vi "Connector Pane Initialization.vi"(8 "error in (no error)":errorcluster, 11 "Data in":T1={"Class"={"Ants"=refnum, "Layer"=refnum, "Templates"=refnum, "Icon"=refnum, "Glyph"=refnum, "Settings"=refnum, "Tools"=refnum, "History"=refnum}, "Ref"={"Add Layer"=refnum, "Remove Layer"=refnum, "Line Text"=[], "Body Text Spec"=refnum, "DNL_Font"=refnum, "glyph path str"=refnum, "templates path str"=refnum, "Arrow Up"=refnum, "Arrow Down"=refnum, "IE VI Ref"=refnum, "Glyphs tree"=refnum, "Templates tree"=refnum, "Layer Icon Text"=refnum, "Layer Template"=refnum, "Body Text"=refnum, "Search Templates"=refnum, "TextMarker"=refnum, "Tab Control"=refnum, "Search Glyphs"=refnum, "Line Color"=refnum, "DNL_Glyphs []"=refnum, "Fill Color"=refnum, "Tools"=refnum, "Icon"=refnum, "Preview"=refnum, "Ants"=refnum, "Terminals"=refnum, "menu reference"=refnum, "LayerNames"=[], "GlyphLoadAnimation"=refnum, "TemplateLoadAnimation"=refnum, "refreshGlyphs"=refnum, "refreshTemplates"=refnum}, "Support"={"AntsRect"={"left"=0, "top"=0, "right"=0, "bottom"=0}, "Mouse Move Coords"={"Horizontal"=0, "Vertical"=0}, "Mouse Down Coords"={"Horizontal"=0, "Vertical"=0}, "Temp Coord"={"Horizontal"=0, "Vertical"=0}, "Action"=enum."Default", "Edge Color"=4914962, "Fill Color"=16860, "Mouse Down?"=FALSE, "Draft Mode?"=FALSE, "Temp Icon"=bytes[3102], "CTRL Pressed"=FALSE, "Move Selection?"=FALSE, "AntsRect Orig"={"left"=0, "top"=0, "right"=0, "bottom"=0}, "Text"="", "TM Set?"=FALSE, "Mouse inside icon?"=FALSE, "Tool (old value)"=0, "Pencil Move Color"=0, "Swap Colors?"=FALSE, "Shift pressed?"=FALSE}}) -> (0 "error out":errorcluster, 3 "Data out":T1={"Class"={"Ants"=refnum, "Layer"=refnum, "Templates"=refnum, "Icon"=refnum, "Glyph"=refnum, "Settings"=refnum, "Tools"=refnum, "History"=refnum}, "Ref"={"Add Layer"=refnum, "Remove Layer"=refnum, "Line Text"=[], "Body Text Spec"=refnum, "DNL_Font"=refnum, "glyph path str"=refnum, "templates path str"=refnum, "Arrow Up"=refnum, "Arrow Down"=refnum, "IE VI Ref"=refnum, "Glyphs tree"=refnum, "Templates tree"=refnum, "Layer Icon Text"=refnum, "Layer Template"=refnum, "Body Text"=refnum, "Search Templates"=refnum, "TextMarker"=refnum, "Tab Control"=refnum, "Search Glyphs"=refnum, "Line Color"=refnum, "DNL_Glyphs []"=refnum, "Fill Color"=refnum, "Tools"=refnum, "Icon"=refnum, "Preview"=refnum, "Ants"=refnum, "Terminals"=refnum, "menu reference"=refnum, "LayerNames"=[], "GlyphLoadAnimation"=refnum, "TemplateLoadAnimation"=refnum, "refreshGlyphs"=refnum, "refreshTemplates"=refnum}, "Support"={"AntsRect"={"left"=0, "top"=0, "right"=0, "bottom"=0}, "Mouse Move Coords"={"Horizontal"=0, "Vertical"=0}, "Mouse Down Coords"={"Horizontal"=0, "Vertical"=0}, "Temp Coord"={"Horizontal"=0, "Vertical"=0}, "Action"=enum."Default", "Edge Color"=4914962, "Fill Color"=16860, "Mouse Down?"=FALSE, "Draft Mode?"=FALSE, "Temp Icon"=bytes[3102], "CTRL Pressed"=FALSE, "Move Selection?"=FALSE, "AntsRect Orig"={"left"=0, "top"=0, "right"=0, "bottom"=0}, "Text"="", "TM Set?"=FALSE, "Mouse inside icon?"=FALSE, "Tool (old value)"=0, "Pencil Move Color"=0, "Swap Colors?"=FALSE, "Shift pressed?"=FALSE}})   [LabVIEW 2020]
uses:
  Class/Ants/Ants.lvclass
  Class/FakedArray/FakedArray.lvclass
  vi.lib/LabVIEW Icon API/lv_icon/Classes/Icon/Icon.lvclass
  Class/Icon Library/Glyph.lvclass
  Class/Settings/Settings.lvclass
  Class/Tools/Tools Paint.lvclass
  <vilib>/Utility/miscctls.llb/LVRectTypeDef.ctl
  <vilib>/Utility/miscctls.llb/LVPoint32TypeDef.ctl
  Controls/SupportClass_Action.ctl
  vi.lib/LabVIEW Icon API/lv_icon/Controls/IEColor.ctl
  Controls/Support Cluster.ctl
  lv_icon.lvlib
  Controls/References Cluster.ctl
  Controls/IE Classes.ctl
  Controls/Global Data.ctl
  History/History/History.lvclass
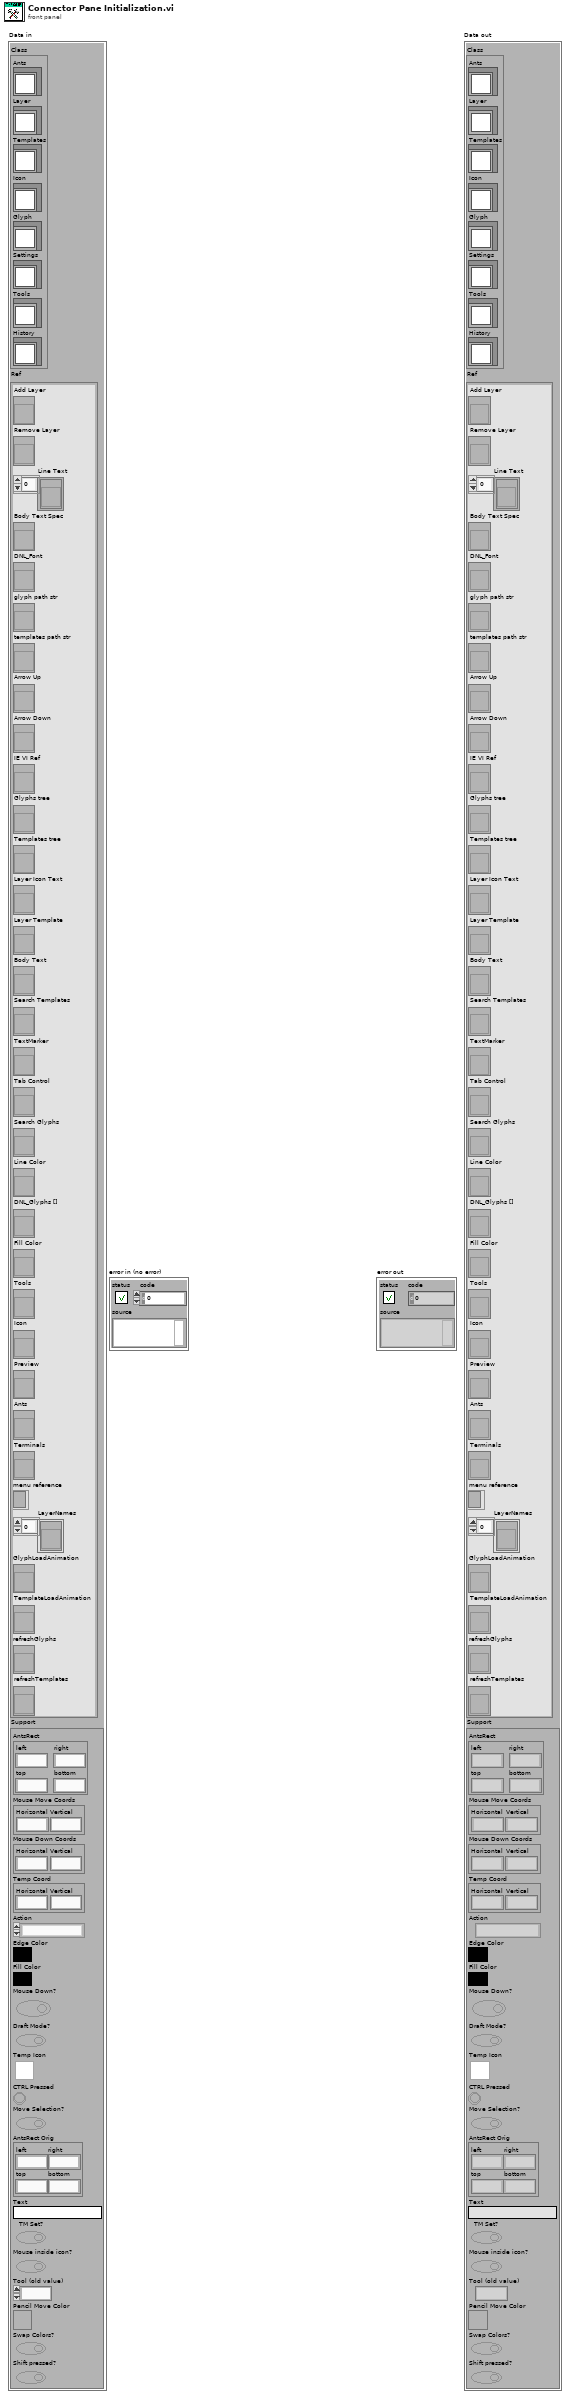
[diagram p1: front panel]
types:
  T1 = typedef "lv_icon.lvlib/Global Data.ctl" = cluster{"Class":T2, "Ref":T3, "Support":T4}
  T2 = typedef "lv_icon.lvlib/IE Classes.ctl" = cluster{"Ants":refnum<class "Ants.lvclass">, "Layer":refnum<class "FakedArray.lvclass">, "Templates":refnum<class "FakedArray.lvclass">, "Icon":refnum<class "Icon.lvclass">, "Glyph":refnum<class "Glyph.lvclass">, "Settings":refnum<class "Settings.lvclass">, "Tools":refnum<class "Tools Paint.lvclass">, "History":refnum<class "History.lvclass">}
  T3 = typedef "lv_icon.lvlib/References Cluster.ctl" = cluster{"Add Layer":refnum<vi>, "Remove Layer":refnum<vi>, "Line Text":refnum<vi>[], "Body Text Spec":refnum<vi>, "DNL_Font":refnum<vi>, "glyph path str":refnum<vi>, "templates path str":refnum<vi>, "Arrow Up":refnum<vi>, "Arrow Down":refnum<vi>, "IE VI Ref":refnum<vi>, "Glyphs tree":refnum<vi>, "Templates tree":refnum<vi>, "Layer Icon Text":refnum<vi>, "Layer Template":refnum<vi>, "Body Text":refnum<vi>, "Search Templates":refnum<vi>, "TextMarker":refnum<vi>, "Tab Control":refnum<vi>, "Search Glyphs":refnum<vi>, "Line Color":refnum<vi>, "DNL_Glyphs []":refnum<vi>, "Fill Color":refnum<vi>, "Tools":refnum<vi>, "Icon":refnum<vi>, "Preview":refnum<vi>, "Ants":refnum<vi>, "Terminals":refnum<vi>, "menu reference":refnum<k9>, "LayerNames":refnum<vi>[], "GlyphLoadAnimation":refnum<vi>, "TemplateLoadAnimation":refnum<vi>, "refreshGlyphs":refnum<vi>, "refreshTemplates":refnum<vi>}
  T4 = typedef "lv_icon.lvlib/Support Cluster.ctl" = cluster{"AntsRect":cluster{"left":i16, "top":i16, "right":i16, "bottom":i16}, "Mouse Move Coords":T5, "Mouse Down Coords":T5, "Temp Coord":T5, "Action":T6, "Edge Color":T7, "Fill Color":T7, "Mouse Down?":bool, "Draft Mode?":bool, "Temp Icon":picture, "CTRL Pressed":bool, "Move Selection?":bool, "AntsRect Orig":cluster{"left":i16, "top":i16, "right":i16, "bottom":i16}, "Text":string, "TM Set?":bool, "Mouse inside icon?":bool, "Tool (old value)":u32, "Pencil Move Color":u32, "Swap Colors?":bool, "Shift pressed?":bool}
  T5 = typedef "LVPoint32TypeDef.ctl" = cluster{"Horizontal":i32, "Vertical":i32}
  T6 = typedef "SupportClass_Action.ctl" = enum16{"Default", "Move Selection", "Glyph Library", "Tool"}
  T7 = typedef "IEColor.ctl" = u32
  T8 = typedef "LVRectTypeDef.ctl" = cluster{"Left":i16, "Top":i16, "Right":i16, "Bottom":i16}
  T9 = typedef "Who Invoked Icon Editor.ctl" = cluster{"Icon Editor Invoker Type":T10, "App Refnum of Invoker":refnum<vi>, "Qualified Name of Invoker":string, "Path to Invoker":path}
  T10 = typedef "Icon Editor Invoker Type.ctl" = enum32{"Unknown Icon Source", "VI Icon", "Library Icon (any library type)", "Palette icon", "Icon from App Method"}
  T11 = enum32{"invalid VI type", "Standard VI", "Control VI", "Global VI", "Polymorphic VI", "Configuration VI", "SubSystem", "Facade VI", "Method VI", "Statechart Diagram VI"}
  T12 = typedef "imagedata.ctl" = cluster{"image type":i32, "image depth":i32, "image":u8[], "mask":u8[], "colors":u32[], "Rectangle":cluster{"left":i16, "top":i16, "right":i16, "bottom":i16}}
  T13 = typedef "lv_icon.lvlib/INI Data.ctl" = cluster{"Show Terminals?":bool, "Text":cluster{"Font":T14, "Alignment":T15, "Size":T16}, "3rd party Templates":cluster{"Store 3rd party Templates?":bool, "Folder Name":string}, "Merge user layers on commit":bool, "Body Text":T17, "Fill Color":T7, "Edge Color":T7, "Tab":u16, "Tool":T18, "Disable Layers?":bool}
  T14 = typedef "Font.ctl" = string
  T15 = typedef "Alignment.ctl" = u16
  T16 = typedef "Font Size.ctl" = u8
  T17 = typedef "BodyText.ctl" = cluster{"Line 1 text":string, "Line 2 text":string, "Line 3 text":string, "Line 4 text":string, "Line 1 color":u32, "Line 2 color":u32, "Line 3 color":u32, "Line 4 color":u32, "Body Text Spec":cluster{"Font":T14, "Alignment":T15, "Size":u8}, "Center text vertically":bool, "Capitalize Text":bool}
  T18 = typedef "Tools.ctl" = enum32{"Pencil", "Line", "Dropper", "Fill", "Rectangle", "Filled Rectangle", "Ellipse", "Filled Ellipse", "Eraser", "Text", "Select", "Move"}
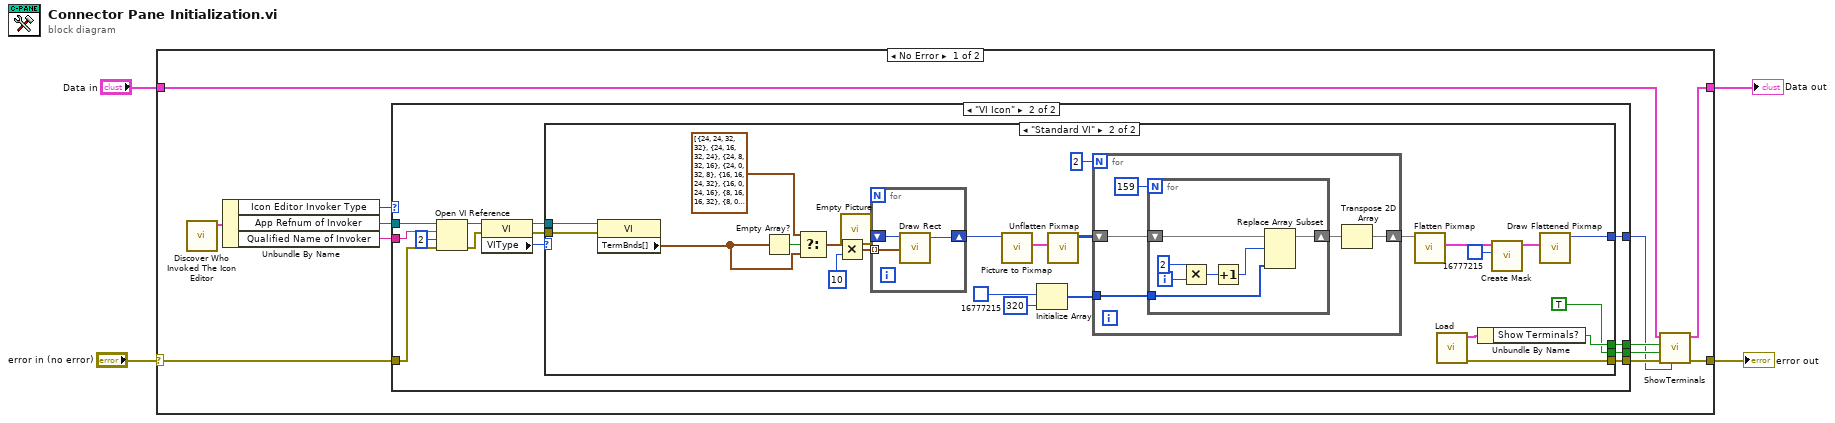
[diagram p0: block diagram]
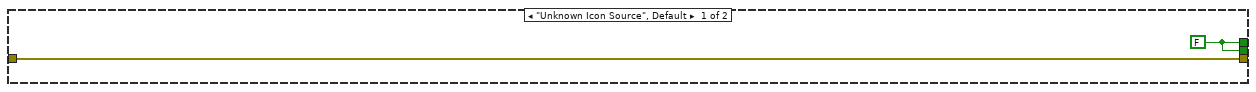
[diagram p2: hidden frame]
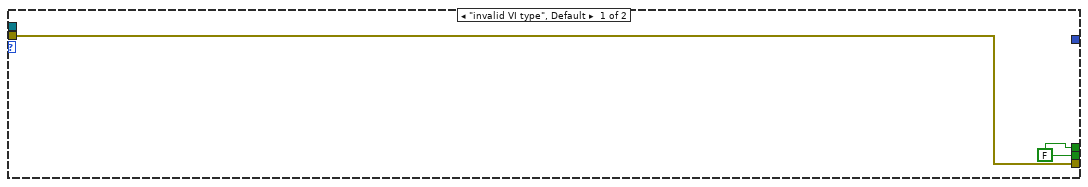
[diagram p3: hidden frame]
diagram:
  n1 = case shown="No Error" "error in (no error)" {
    selector: "error in (no error)" -> [w11 w75]
    tunnel: [w16 w75] -> w3
    tunnel: "Data in" -> [w7 w74]
    tunnel: [w6 w74] -> w1
    frame No Error {
      n2 = call <resource>:"Discover Who Invoked The Icon Editor.vi"() -> ("Who Invoked The Icon Editor?"=w14:T9)  [unwired: 11 out]
      n3 = Unbundle By Name(w14) -> ("Icon Editor Invoker Type"=w9:T10, "App Refnum of Invoker"=w13:refnum<vi>, "Qualified Name of Invoker"=w12:string)
      n4 = case shown="\"VI Icon\"" w9 {
        tunnel: [w18 w31] -> w15
        tunnel: w13 -> [_ w30]
        tunnel: w12 -> [_ w29]
        tunnel: w11 -> [w17 w28]
        tunnel: [w17 w27] -> w10
        tunnel: [w18 w26] -> w8
        tunnel: [_ w20] -> w5
        frame "Unknown Icon Source", Default {
          w18 = FALSE
        }
        frame "VI Icon" {
          n5 = Open VI Reference(application reference (local)=w30, vi path=w29, options=2, error in (no error)=w28) -> (vi reference=w22:refnum<vi>, error out=w23:errorcluster)  [unwired: 2 out]
          n6 = property class="VI"(reference=w22, error in=w23) -> (reference out=w25:refnum<vi>, error out=w24:errorcluster, "VIType"=w21:T11)
          n7 = case shown="\"Standard VI\"" w21 {
            tunnel: [w32 w57] -> w31
            tunnel: [w33 w56] -> w27
            tunnel: [w32 TRUE] -> w26
            tunnel: w25 -> [_ w36]
            tunnel: w24 -> [w33 w35]
            tunnel: [_ w43] -> w20
            frame "invalid VI type", Default {
              w32 = FALSE
            }
            frame "Standard VI" {
              n8 = property class="VI"(reference=w36, error in=w35) -> ("TermBnds[]"=w34:T8[])  [unwired: 2 out]
              n9 = Empty Array?(array=w34) -> (empty?=w42:bool)
              n10 = Select(t=T8[] [{"Left"=24, "Top"=24, "Right"=32, "Bottom"=32}, {"Left"=24, "Top"=16, "Right"=32, "Bottom"=24}, {"Left"=24, "Top"=8, "Right"=32, "Bottom"=16}, {"Left"=24, "Top"=0, "Right"=32, "Bottom"=8}, {"Left"=16, "Top"=16, "Right"=24, "Bottom"=32}, {"Left"=16, "Top"=0, "Right"=24, "Bottom"=16}, {"Left"=8, "Top"=16, "Right"=16, "Bottom"=32}, {"Left"=8, "Top"=0, "Right"=16, "Bottom"=16}, {"Left"=0, "Top"=24, "Right"=8, "Bottom"=32}, {"Left"=0, "Top"=16, "Right"=8, "Bottom"=24}, {"Left"=0, "Top"=8, "Right"=8, "Bottom"=16}, {"Left"=0, "Top"=0, "Right"=8, "Bottom"=8}] ("Terminal Bounds[]"), s=w42, f=w34) -> (s? t:f=w41:T8[])
              n11 = Multiply(x=w41, y=i16 10) -> (x*y=w45:T8[])
              n12 = call "Empty Picture"() -> ("empty picture"=w46:picture)
              n13 = for {
                tunnel: w45 -> [w73] mode=indexing
                shift-right: [w72] -> w47
                shift-left: w46 -> [w71]
                n14 = call <vilib>:"Draw Rect.vi"("picture"=w71, "rect"=w73) -> ("new picture"=w72:picture)  [unwired: 7 in]
              }
              n15 = call <vilib>:"Picture to Pixmap.vi"("picture"=w47) -> ("image data"=w48:T12)  [unwired: 9 in, 1 out]
              n16 = Initialize Array(u32 16777215, 320 ("dimension size")) -> (w53:u32[])
              n17 = call <vilib>:"Unflatten Pixmap.vi"("image data"=w48) -> ("24-bit pixmap"=w49:u32[][])  [unwired: 4 in, 6 out]
              n18 = for {
                N: 2 -> [_]
                shift-right: [w61] -> w54
                shift-left: w49 -> [w63]
                tunnel: w53 -> [w59]
                n19 = for {
                  N: 159 -> [_]
                  shift-right: [w65] -> w62
                  shift-left: w63 -> [w70]
                  tunnel: w59 -> [w64]
                  i -> [w69]
                  n20 = Multiply(x=2, y=w69) -> (x*y=w68:i32)
                  n21 = Increment(x=w68) -> (x+1=w66:i32)
                  n22 = Replace Array Subset(array=w70, new element=w64, index (row)=w66) -> (w65:u32[][])  [unwired: 1 in]
                }
                n23 = Transpose 2D Array(2D array=w62) -> (transposed array=w61:u32[][])
              }
              n24 = call <vilib>:"Flatten Pixmap.vi"("24-bit pixmap"=w54) -> ("image data"=w39:T12)  [unwired: 10 in]
              n25 = call "Load.vi"() -> ("error out"=w56:errorcluster, "INI Data"=w58:T13)  [unwired: 3 in, 7 out]
              n26 = Unbundle By Name(w58) -> ("Show Terminals?"=w57:bool)
              n27 = call <vilib>:"Create Mask.vi"("Mask Color (Black)"=u32 16777215, "image data"=w39) -> ("image data"=w38:T12)  [unwired: 9 in]
              n28 = call <vilib>:"Draw Flattened Pixmap.vi"("image data"=w38) -> ("new picture"=w43:picture)  [unwired: 8 in]
            }
          }
        }
      }
      n29 = call "ShowTerminals.vi"("LayerIcon"=w5, "error in"=w10, "Tag enabled?"=w8, "Show Terminals?"=w15, "Data in"=w7) -> ("error out"=w16:errorcluster, "Data out"=w6:T1)  [unwired: 1 in, 4 out]
    }
    frame Error {
    }
  }
  "error out" <- w3
  "Data out" <- w1
